vi "Configure Measurement Edge (Threshold).vi"(5 "Threshold Lower Value (10.0 %)":dbl=10.0, 7 "Threshold Middle Value (50.0 %)":dbl=50.0, 8 "error in (no error)":errorcluster, 9 "Threshold Upper Value (90.0 %)":dbl=90.0, 10 "Threshold Type (0: Standard)":i32(ring) items=["Standard", "Percent", "Absolute"], 11 "VISA resource name":refnum<visa-resource-name>) -> (0 "error out":errorcluster, 3 "VISA resource name out":refnum<visa-resource-name>)   [LabVIEW 2015, in "Agilent 2000 3000 X-Series.lvlib"]
doc: "Configure the edge threshold in measurement."
uses:
  Agilent 2000 3000 X-Series.lvlib
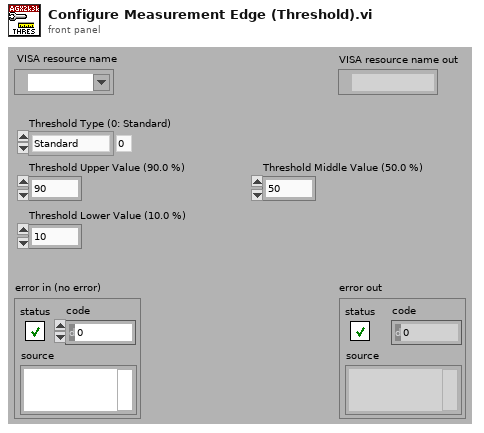
[diagram p1: front panel]
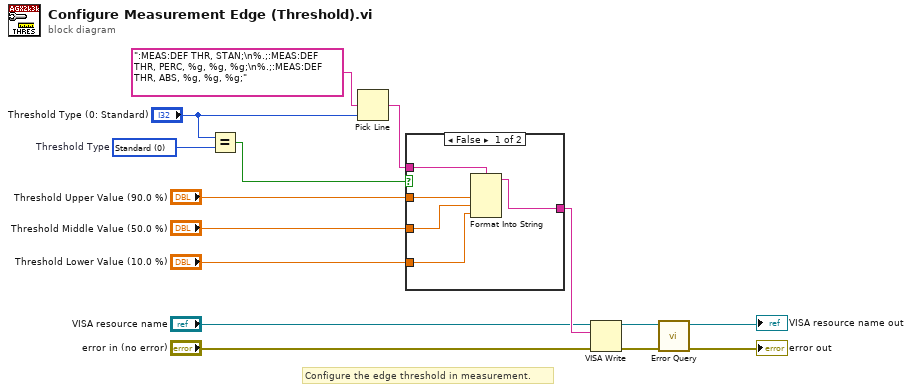
[diagram p0: block diagram]
diagram:
  w2 = 0 items=["Standard", "Percent", "Absolute"]  # Threshold Type
  # "Configure the edge threshold in measurement."
  n1 = Equal?(x="Threshold Type (0: Standard)", y=w2) -> (x = y?=w12:bool)
  n2 = Pick Line(multi-line string=":MEAS:DEF THR, STAN;\n%.;:MEAS:DEF THR, PERC, %g, %g, %g;\n%.;:MEAS:DEF THR, ABS, %g, %g, %g;", line index="Threshold Type (0: Standard)") -> (output string=w10:string)  [unwired: 1 out]
  n3 = case shown="False" w12 {
    tunnel: "Threshold Lower Value (10.0 %)" -> [w16 _]
    tunnel: "Threshold Middle Value (50.0 %)" -> [w17 _]
    tunnel: "Threshold Upper Value (90.0 %)" -> [w18 _]
    tunnel: [w20 w21] -> w9
    tunnel: w10 -> [w19 w21]
    frame False {
      n4 = Format Into String(format string=w19, w18, w17, w16) -> (resulting string=w20:string)  [unwired: 2 in, 1 out]
    }
    frame True {
    }
  }
  n5 = VISA Write(VISA resource name="VISA resource name", write buffer=w9, error in (no error)="error in (no error)") -> (VISA resource name out=w8:refnum<visa-resource-name>, error out=w5:errorcluster)  [unwired: 1 out]
  n6 = call "Error Query.vi"("error in (no error)"=w5, "VISA resource name"=w8) -> ("error out"=→"error out":errorcluster, "VISA resource name out"=→"VISA resource name out":refnum<visa-resource-name>)  [unwired: 8 out]
